vi "file operration exp.vi"() -> ()   [LabVIEW 2024]
panel:
  in  "Controller":bool
  in  "Destination path or location":path
  in  "Source path or loaction":path
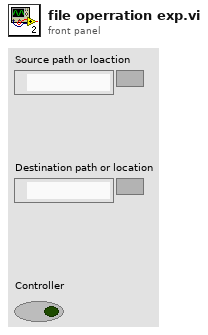
[diagram p1: front panel]
types:
  T1 = enum16{"open", "replace", "create", "open or create", "replace or create", "replace or create with confirmation"}
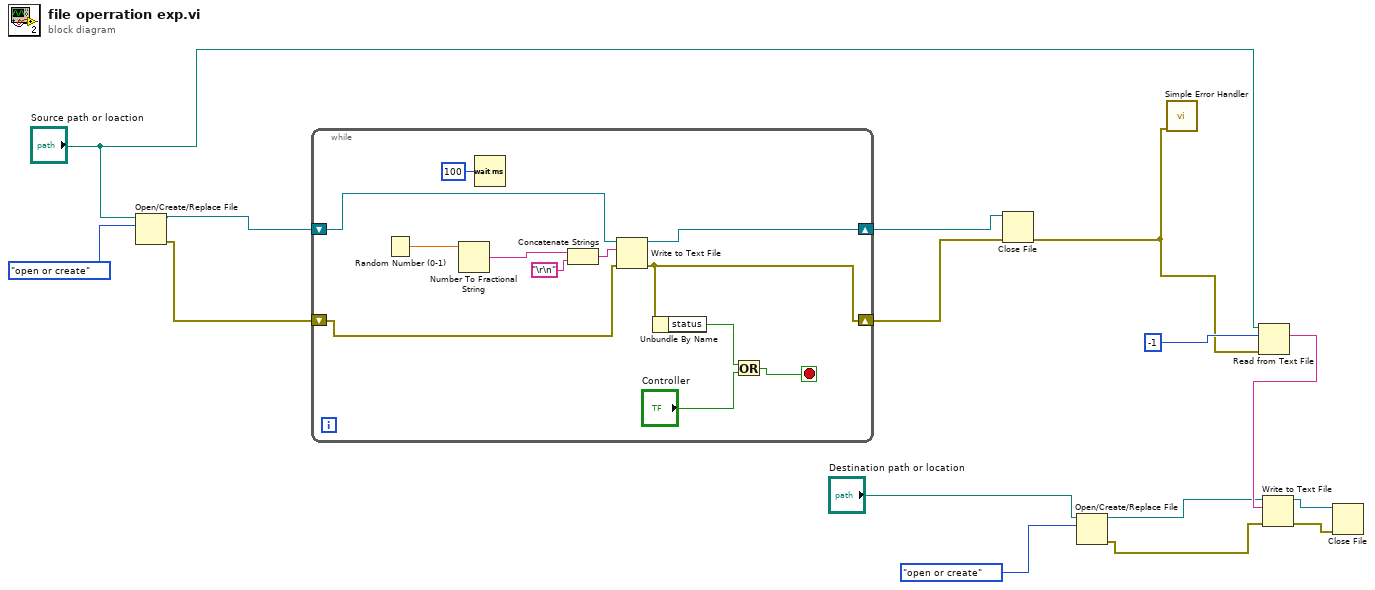
[diagram p0: block diagram]
diagram:
  n1 = Open/Create/Replace File(file path (use dialog)="Source path or loaction", operation (0:open)=T1."open or create") -> (refnum out=w12:refnum<file>, error out=w14:errorcluster)  [unwired: 4 in, 1 out]
  n2 = while {
    shift-right: [w22] -> w11
    shift-left: w12 -> [w23]
    shift-right: [w17] -> w13
    shift-left: w14 -> [w21]
    stop <- w25 stop-if-true
    n3 = Random Number (0-1)() -> (number: 0 to 1=w26:dbl)
    n4 = Number To Fractional String(number=w26) -> (F-format string=w20:string)  [unwired: 3 in]
    n5 = Wait (ms)(milliseconds to wait=u32 100) -> ()  [unwired: 1 out]
    n6 = Concatenate Strings(w20, "\r\n") -> (w24:string)
    n7 = Write to Text File(file (use dialog)=w23, text=w24, error in=w21) -> (refnum out=w22:refnum<file>, error out=w17:errorcluster)  [unwired: 1 in, 1 out]
    n8 = Unbundle By Name(w17) -> ("status"=w18:bool)
    n9 = Or(x=w18, y="Controller") -> (x .or. y?=w25:bool)
  }
  n10 = Close File(refnum=w11, error in=w13) -> (error out=w3:errorcluster)  [unwired: 1 out]
  n11 = Open/Create/Replace File(file path (use dialog)="Destination path or location", operation (0:open)=T1."open or create") -> (refnum out=w7:refnum<file>, error out=w5:errorcluster)  [unwired: 4 in, 1 out]
  n12 = call <vilib>:"Simple Error Handler.vi"("error in (no error)"=w3) -> ()  [unwired: 4 in, 5 out]
  n13 = Read from Text File(file (use dialog)="Source path or loaction", count=-1, error in=w3) -> (text=w8:string)  [unwired: 1 in, 3 out]
  n14 = Write to Text File(file (use dialog)=w7, text=w8, error in=w5) -> (refnum out=w6:refnum<file>, error out=w4:errorcluster)  [unwired: 1 in, 1 out]
  n15 = Close File(refnum=w6, error in=w4) -> ()  [unwired: 2 out]
